vi "33_Basics of Bundle and Unbundle.vi"() -> ()   [LabVIEW 2018]
panel:
  out "Gender 2":bool
  out "Age 2":dbl
  out "Last Name 2":string
  out "First Name 2":string
  in  "Cluster 2":T1
  out "Gender":bool
  out "Age":dbl
  out "Last Name":string
  out "First Name":string
  in  "Cluster":T2
  # "Unbulde By name"
  # "Unbundle"
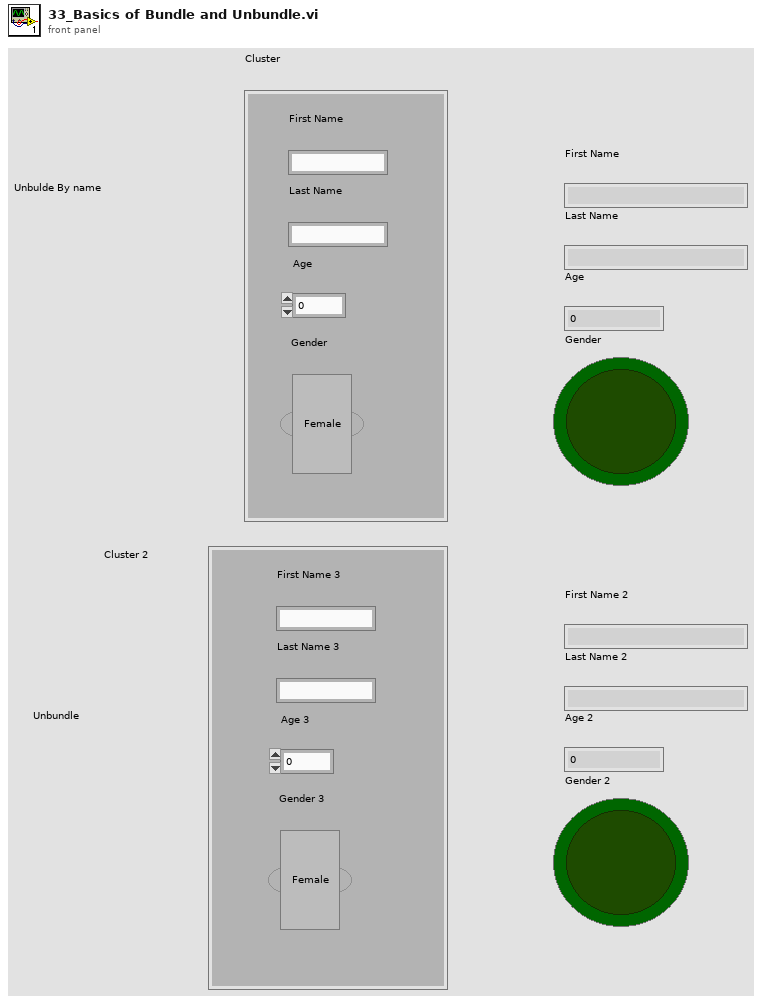
[diagram p1: front panel]
types:
  T1 = cluster{"First Name 3":string, "Last Name 3":string, "Age 3":dbl, "Gender 3":bool}
  T2 = cluster{"First Name":string, "Last Name":string, "Age":dbl, "Gender":bool}
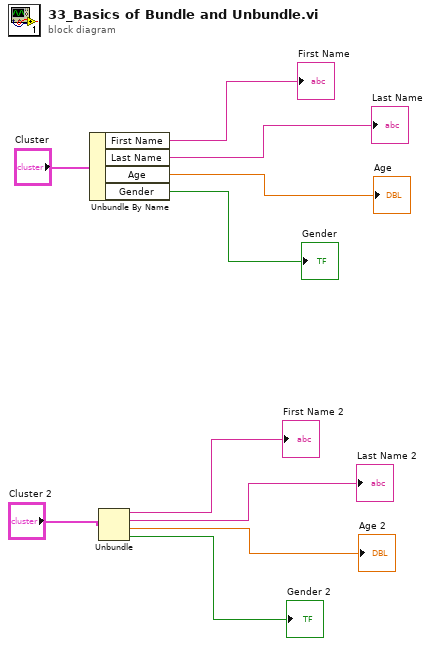
[diagram p0: block diagram]
diagram:
  n1 = Unbundle By Name("Cluster") -> ("First Name"=→"First Name":string, "Last Name"=→"Last Name":string, "Age"=→"Age":dbl, "Gender"=→"Gender":bool)
  n2 = Unbundle("Cluster 2") -> ("First Name 3"=→"First Name 2":string, "Last Name 3"=→"Last Name 2":string, "Age 3"=→"Age 2":dbl, "Gender 3"=→"Gender 2":bool)
